vi "PCO_CloseCamera.vi"(8 "error in (no error)":errorcluster {"code" format="%x"}, 11 "ph":u64) -> (0 "error out":errorcluster {"code" format="%x"}, 2 "ErrorMessage":i32 format="%x")   [LabVIEW 2019, in "SDK.lvlib" / "CameraAccess.lvlib"]
doc: "<b>Description:</b>\nThis function is used to close the connection to a previously opened camera.\n\n<b>Supported camera type:</b>\nAll cameras\n\n<b>Descriptor dependency:</b>\nNone"
uses:
  CameraAccess.lvlib
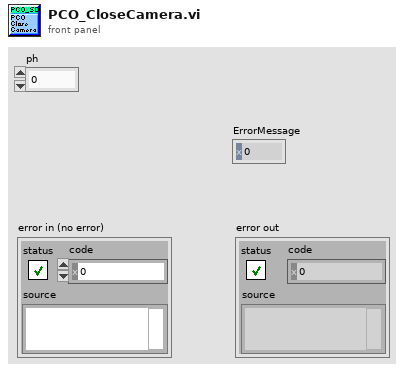
[diagram p1: front panel]
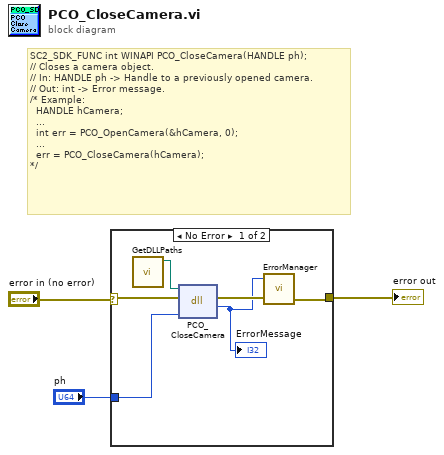
[diagram p0: block diagram]
diagram:
  # "SC2_SDK_FUNC int WINAPI PCO_CloseCamera(HANDLE ph);\n// Closes a camera object.\n// In: HANDLE ph -> Handle to a previously opened camera.\n// Out: int -> Error message.\n/* Example:\n  HANDLE hCamera;\n  ...\n  int err = PCO_OpenCamera(&hCamera, 0);\n  ...\n  err = PCO_CloseCamera(hCamera);\n*/"
  n1 = case shown="No Error" "error in (no error)" {
    selector: "error in (no error)" -> [w5 w10]
    tunnel: [w8 w10] -> w3
    tunnel: "ph" -> [w6 _]
    frame No Error {
      n2 = call "GetDLLPaths.vi"() -> ("SC2_Cam_Path"=w4:path)  [unwired: 8 in, 3 out]
      n3 = dll-call lib="?" fn="PCO_CloseCamera"(path in=w4, error in=w5, "ph"=w6) -> (error out=w9:errorcluster, "return type"=w7:i32)  [unwired: 2 in, 1 out]
      "ErrorMessage" <- w7
      n4 = call "ErrorManager.vi"("error in (no error)"=w9, "error code"=w7) -> ("error out"=w8:errorcluster)  [unwired: 2 in, 1 out]
    }
    frame Error {
    }
  }
  "error out" <- w3
